vi "hp34401 multimetro status.vi"() -> ()   [LabVIEW 2012]
panel:
  in  "String":string
  out "byte count":i32
  out "error code":string="0\tEDVR\tError connecting to driver.\n1\tECIC\tCommand requires GPIB Controller to be CIC.\n2\tENOL\tWrite detected no Listeners.\n3\tEADR\tGPIB Controller not addressed correctly.\n4\tEARG\tInvalid argument or arguments.\n5\tESAC\tCommand requires GPIB Controller to be SC.\n6\tEABO\tI/O operation aborted.\n7\tENEB\tNon-existent board.\n8\tEDMA\tDMA Hardware error detected.\n9\tEBTO\tDMA hardware mP bus timeout.\n11\tECAP\tNo capability.\n12\tEFSO\tFile system operation error.\n13\tEOWN\tShareable board exclusively owned.\n14\tEBUS\tGPIB bus error.\n15\tESTB\tSerial poll byte queue overflow.\n16\tESRQ\tSRQ stuck on.\n17\tECMD\tUnrecognized command.\n19\tEBNP\tBoard not present.\n20\tETAB\tTable error.\n30\tNADDR\tNo GPIB address input.\n31\tNSTRG\tNo string input (write).\n32\tNCNT\tNo count input (read)."
  out "GPIB error code":i16
  out "GPIB status out":bool[](array[boolean])
  out "status after read":bool[](array[boolean])
  out "status after \nwrite: read?":bool[](array[boolean])
  out "status after write 1":bool[](array[boolean])
  out "status vector":string="Status Bits Table\n\nStatus Bit \tNumericValue\t Symbolic Status\tDescription\n0\t              1\t                      DCAS\tDevice Clear state\n1\t              2\t                      DTAS\tDevice Trigger State\n2\t              4\t                      LACS\tListener Active\n3\t              8\t                      TACS\tTalker Active\n4\t              16\t                     ATN\tAttention Asserted\n5\t              32\t                     CIC\tController-In-Charge\n6\t              64\t                     REM\tRemote State\n7\t              128\t                   LOK\tLockout State\n8\t              256\t                   CMPL\tOperation Completed\n12\t            4096\t                 SRQI\tSRQ Detected while CIC\n13            \t8192                  END\tEOI or EOS Detected\n14\t            16384\t               TIMO\tTimeout\n15\t            -32768\t              ERR\tError Detected\n"
  out "Tensione":dbl format="%.8f"
  out "Valore di tensione":string
  # "Registro di STATO della Scheda GPIB durante la\nconfigurazione del multimetro (conf:volt:ac), la lettura  del dato (:read?), etc."
  # "Si riferisce al controller"
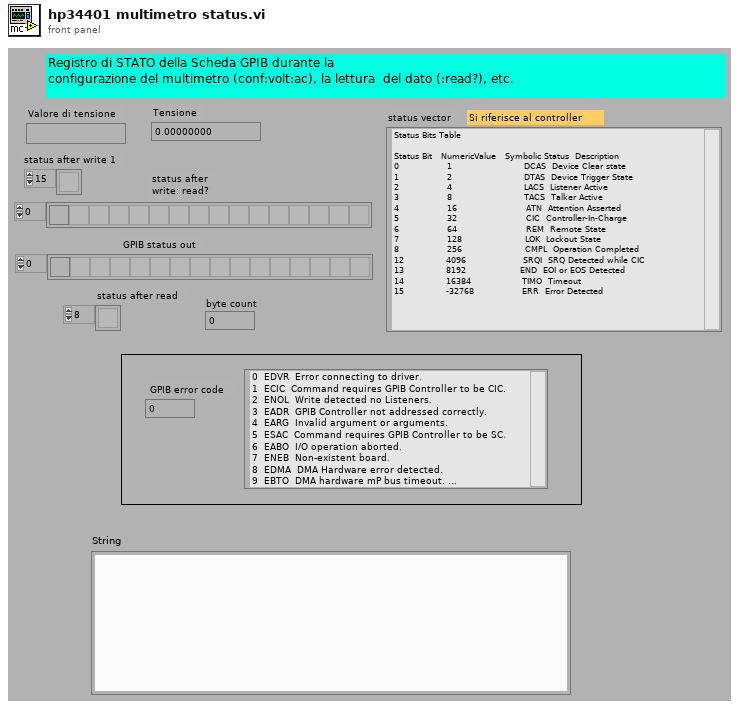
[diagram p1: front panel]
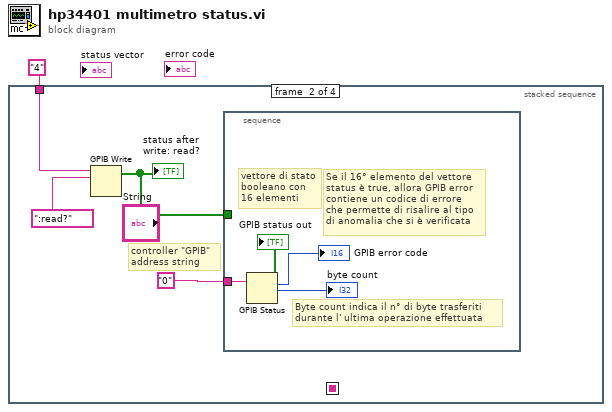
[diagram p0: block diagram]
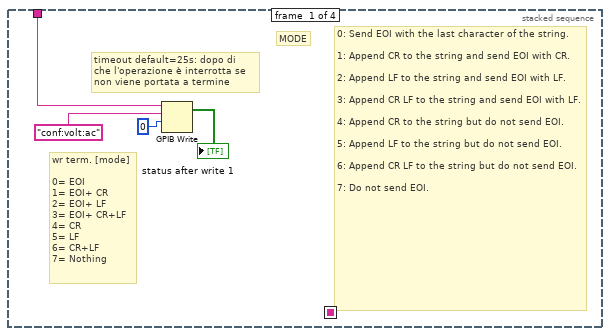
[diagram p2: hidden frame]
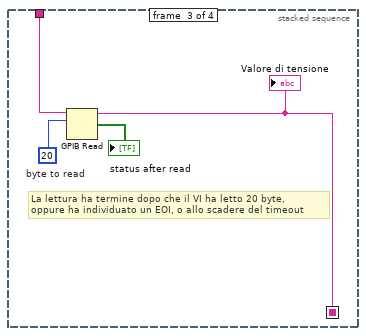
[diagram p3: hidden frame]
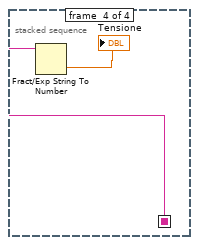
[diagram p4: hidden frame]
diagram:
  n1 = stacked-sequence {
    seq-local: [_ _ w14 _] -> [_ _ _ w18]
    tunnel: "4" -> [w4 w8 w16 _]
    frame #0 {
      # "wr term. [mode]\n\n0= EOI\n1= EOI+ CR\n2= EOI+ LF\n3= EOI+ CR+LF\n4= CR\n5= LF\n6= CR+LF\n7= Nothing"
      # "0:\tSend EOI with the last character of the string.\n\n1:\tAppend CR to the string and send EOI with CR.\n\n2:\tAppend LF to the string and send EOI with LF.\n\n3:\tAppend CR LF to the string and send EOI with LF.\n\n4:\tAppend CR to the string but do not send EOI.\n\n5:\tAppend LF to the string but do not send EOI.\n\n6:\tAppend CR LF to the string but do not send EOI.\n\n7:\tDo not send EOI."
      # "MODE"
      # "timeout default=25s: dopo di \nche l'operazione è interrotta se\nnon viene portata a termine"
      n2 = GPIB Write(0:w4, 1:"conf:volt:ac", 2:i16 0 ("mode (0)")) -> (5:→"status after write 1":bool[])  [unwired: 2 in, 1 out]
    }
    frame #1 {
      # "controller \"GPIB\" \naddress string"
      n3 = GPIB Write(0:w8, 1:":read?") -> (5:w7:bool[])  [unwired: 3 in, 1 out]
      "status after \nwrite: read?" <- w7
      n4 = stacked-sequence {
        tunnel: w7 -> [_]
        tunnel: "0" -> [w13]
        frame #0 {
          # "Byte count indica il n° di byte trasferiti\ndurante l' ultima operazione effettuata"
          # "Se il 16° elemento del vettore\nstatus è true, allora GPIB error\ncontiene un codice di errore\nche permette di risalire al tipo\ndi anomalia che si è verificata"
          # "vettore di stato\nbooleano con\n16 elementi"
          n5 = GPIB Status(0:w13) -> (2:→"GPIB status out":bool[], 3:→"GPIB error code":i16, 4:→"byte count":i32)  [unwired: 1 in, 1 out]
        }
      }
    }
    frame #2 {
      w17 = 20  # byte to read
      # "La lettura ha termine dopo che il VI ha letto 20 byte,\noppure ha individuato un EOI, o allo scadere del timeout"
      n6 = GPIB Read(0:w16, 1:w17) -> (5:w14:string, 6:→"status after read":bool[])  [unwired: 3 in, 1 out]
      "Valore di tensione" <- w14
    }
    frame #3 {
      n7 = Fract/Exp String To Number(string=w18) -> (number=→"Tensione":dbl)  [unwired: 3 in, 1 out]
    }
  }
